vi "Begin.vi"(11 "Image Size":T1=enum."160x120") -> (0 "error out":errorcluster)   [LabVIEW 2012]
doc: "Called before other user functions, this VI is expected to open initial I/O refnums, load in file data, and do all program initialization. Notice that the <B>error out</B> terminal is simply used for data flow. Wiring it to other structures or subVIs ensures that this VI runs first."
uses:
  <vilib>/Rock Robotics/WPI/Camera/WPI_CameraImageSize.ctl
  <vilib>/Rock Robotics/WPI/Camera/WPI_CameraWhite Balance Values.ctl
  <vilib>/Rock Robotics/WPI/Camera/WPI_CameraExposure Values.ctl
  <vilib>/Rock Robotics/WPI/Camera/WPI_CameraFrameRate.ctl
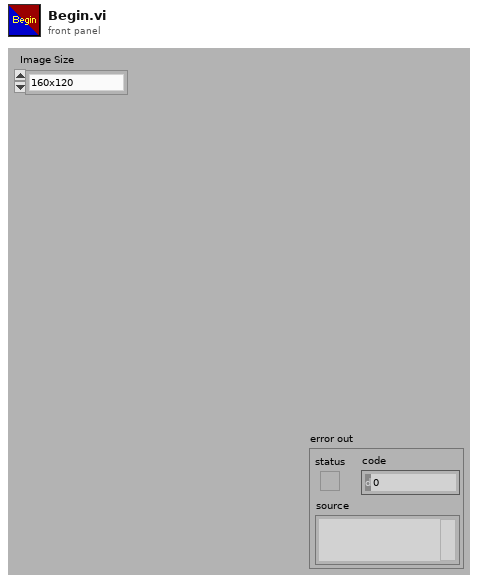
[diagram p1: front panel]
types:
  T1 = typedef "WPI_CameraImageSize.ctl" = enum16{"640x480", "320x240", "160x120"}
  T2 = typedef "WPI_CameraFrameRate.ctl" = u32
  T3 = typedef "WPI_CameraExposure Values.ctl" = enum16{"Auto", "Flicker-free 50 Hz", "Flicker-free 60 Hz", "Hold current"}
  T4 = typedef "WPI_CameraWhite Balance Values.ctl" = enum16{"Auto", "Fixed indoor", "Fixed outdoor 1", "Fixed outdoor 2", "Fixed fluorescent 1", "Fixed fluorescent 2", "Hold current"}
  T5 = typedef "WPI_CameraDevRef.ctl" = cluster{"Camera Address":string, "CameraStatus":errorcluster, "Acquire Image Notifier":refnum<notifier>}
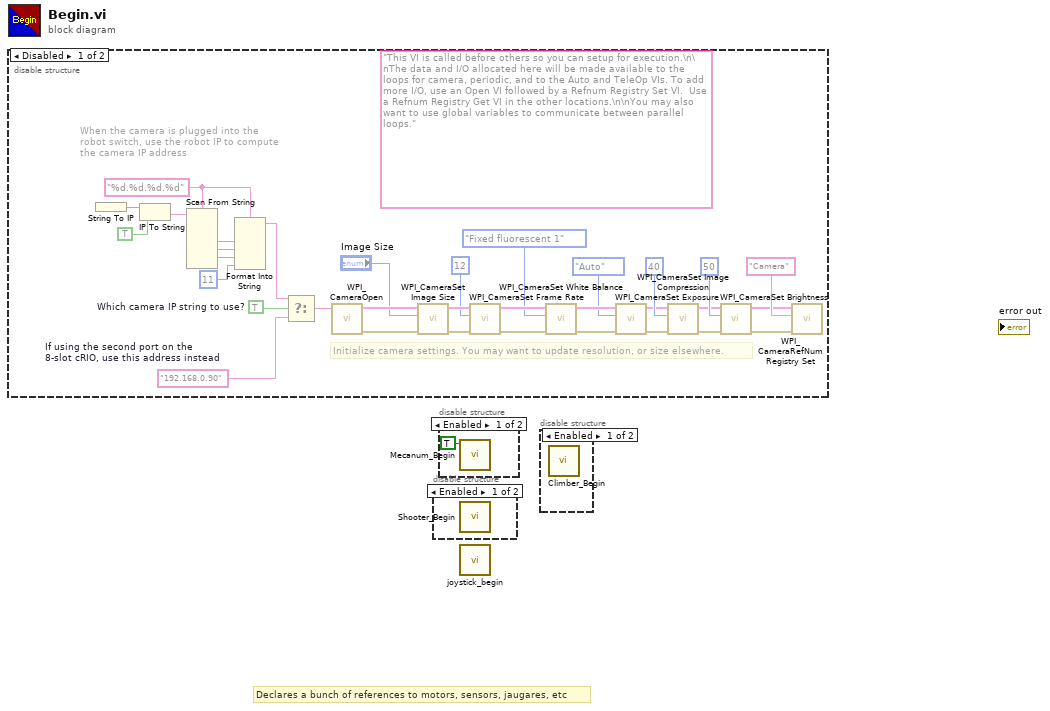
[diagram p0: block diagram]
diagram:
  # "Declares a bunch of references to motors, sensors, jaugares, etc"
  n1 = disable-structure shown="Disabled" {
    frame Disabled {
      w1 = TRUE  # Which camera IP string to use?
      w5 = "%d.%d.%d.%d" ("format string")
      (unwired) "This VI is called before others so you can setup for execution.\n\nThe data and I/O allocated here will be made available to the loops for camera, periodic, and to the Auto and TeleOp VIs. To add more I/O, use an Open VI followed by a Refnum Registry Set VI.  Use a Refnum Registry Get VI in the other locations.\n\nYou may also want to use global variables to communicate between parallel loops."
      w2 = "192.168.0.90"  # If using the second port on the 8-slot cRIO, use this address instead
      # "When the camera is plugged into the\nrobot switch, use the robot IP to compute\nthe camera IP address"
      # "Initialize camera settings. You may want to update resolution, or size elsewhere."
      n2 = String To IP() -> (0:w12:u32)  [unwired: 1 in]
      n3 = IP To String(1:TRUE ("dot notation? (F)"), 2:w12) -> (0:w10:string)
      n4 = Scan From String(format string=w5, input string=w10) -> (output 1=w9:i32, output 2=w8:i32, output 3=w7:i32)  [unwired: 7 in, 3 out]
      n5 = Format Into String(format string=w5, w9, w8, w7, 11 ("Compression")) -> (resulting string=w3:string)  [unwired: 2 in, 1 out]
      n6 = Select(t=w3, s=w1, f=w2) -> (s? t:f=w4:string)
      n7 = call <vilib>:"WPI_CameraOpen.vi"("Camera Address"=w4) -> ("error out"=w24:errorcluster, "CameraDevRef"=w25:T5)  [unwired: 1 in, 8 out]
      n8 = call <vilib>:"WPI_CameraSet Image Size.vi"("error in (no error)"=w24, "Image Size"="Image Size", "CameraDevRef"=w25) -> ("error out"=w23:errorcluster, "CameraDevRef Out"=w26:T5)  [unwired: 7 out]
      n9 = call <vilib>:"WPI_CameraSet Frame Rate.vi"("error in (no error)"=w23, "Frame Rate (fps)"=T2 12, "CameraDevRef"=w26) -> ("error out"=w22:errorcluster, "CameraDevRef Out"=w28:T5)  [unwired: 7 out]
      n10 = call <vilib>:"WPI_CameraSet White Balance.vi"("error in (no error)"=w22, "White Balance"=WPI_CameraWhite_Balance_Values."Fixed fluorescent 1", "CameraDevRef"=w28) -> ("error out"=w21:errorcluster, "CameraDevRef Out"=w27:T5)  [unwired: 7 out]
      n11 = call <vilib>:"WPI_CameraSet Exposure.vi"("error in (no error)"=w21, "Exposure"=WPI_CameraExposure_Values."Auto", "CameraDevRef"=w27) -> ("error out"=w20:errorcluster, "CameraDevRef Out"=w30:T5)  [unwired: 7 out]
      n12 = call <vilib>:"WPI_CameraSet Image Compression.vi"("error in (no error)"=w20, "Compression"=40, "CameraDevRef"=w30) -> ("error out"=w19:errorcluster, "CameraDevRef Out"=w29:T5)  [unwired: 7 out]
      n13 = call <vilib>:"WPI_CameraSet Brightness.vi"("error in (no error)"=w19, "Brightness"=50, "CameraDevRef"=w29) -> ("error out"=w17:errorcluster, "CameraDevRef Out"=w18:T5)  [unwired: 7 out]
      n14 = call <vilib>:"WPI_CameraRefNum Registry Set.vi"("error in (no error)"=w17, "refnum name"="Camera", "CameraDevRef"=w18) -> ()  [unwired: 9 out]
    }
    frame Enabled {
    }
  }
  n15 = disable-structure shown="Enabled" {
    frame Enabled {
      n16 = call "Shooter_Begin.vi"() -> ()  [unwired: 12 in]
    }
    frame Disabled {
    }
  }
  n17 = disable-structure shown="Enabled" {
    frame Enabled {
      n18 = call "Mecanum_Begin.vi"("Brake?"=TRUE) -> ()  [unwired: 11 in]
    }
    frame Disabled {
    }
  }
  n19 = call "joystick_begin.vi"() -> ()  [unwired: 11 in, 1 out]
  n20 = disable-structure shown="Enabled" {
    frame Enabled {
      n21 = call "Climber_Begin.vi"() -> ()  [unwired: 12 in]
    }
    frame Disabled {
    }
  }
